vi "Init User Info List.vi"(8 "error in (no error)":errorcluster, 11 "[V] User List in":refnum<class "[V] User List.lvclass">) -> (0 "error out":errorcluster, 3 "[V] User List out":refnum<class "[V] User List.lvclass">)   [LabVIEW 2020, in "[V] User List.lvlib" / "[V] User List.lvclass"]
uses:
  [V] User List.lvclass
  [V] User List.lvclass/[V] User List.ctl
  <vilib>/Utility/miscctls.llb/LVRowAndColumnTypeDef.ctl
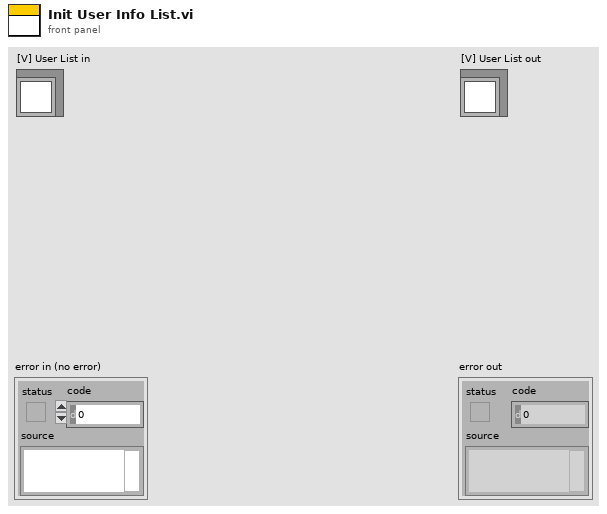
[diagram p1: front panel]
types:
  T1 = typedef "LVRowAndColumnTypeDef.ctl" = cluster{"Row":i32, "Column":i32}
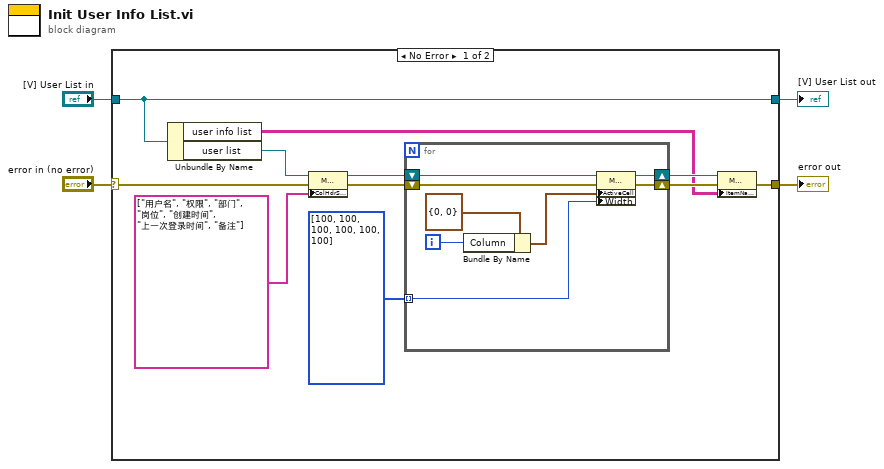
[diagram p0: block diagram]
diagram:
  n1 = case shown="No Error" "error in (no error)" {
    selector: "error in (no error)" -> [w14 w25]
    tunnel: [w6 w25] -> w3
    tunnel: [w15 w24] -> w1
    tunnel: "[V] User List in" -> [w15 w24]
    frame No Error {
      n2 = Unbundle By Name(w15) -> ("user info list"=w7:string[][], "user list"=w13:refnum<vi>)
      n3 = property class="MCListbox (strict)"(reference=w13, error in=w14, "ColHdrString"=string[] ["用户名", "权限", "部门", "岗位", "创建时间", "上一次登录时间", "备注"] ("Column Header Strings[]")) -> (reference out=w10:refnum<vi>, error out=w11:errorcluster)
      n4 = for {
        shift-right: [w18] -> w9
        shift-left: w11 -> [w23]
        shift-right: [w17] -> w8
        shift-left: w10 -> [w22]
        tunnel: u32[] [100, 100, 100, 100, 100, 100] ("Active Cell:Cell Size:Width") -> [w16] mode=indexing
        i -> [w20]
        n5 = Bundle By Name(cluster=T1 {"Row"=0, "Column"=0} ("Active Cell:Active Cell"), "Column"=w20) -> (w19:T1)
        n6 = property class="MCListbox (strict)"(reference=w22, error in=w23, "ActiveCell"=w19, "Width"=w16) -> (reference out=w17:refnum<vi>, error out=w18:errorcluster)
      }
      n7 = property class="MCListbox (strict)"(reference=w8, error in=w9, "ItemNames"=w7) -> (error out=w6:errorcluster)  [unwired: 1 out]
    }
    frame Error {
    }
  }
  "error out" <- w3
  "[V] User List out" <- w1
